vi "Bundle AOL parameters at start.vi"(6 "Case name string":string, 8 "error in (no error)":errorcluster) -> (0 "error out":errorcluster, 2 "cancelled":bool)   [LabVIEW 2013]
uses:
  Typedefs/Imaging Protocols enum.ctl
  Typedefs/AOL modes.ctl
  Global Variables/gl_UI Ctrl Refs.vi
  Global Variables/General Globals.vi
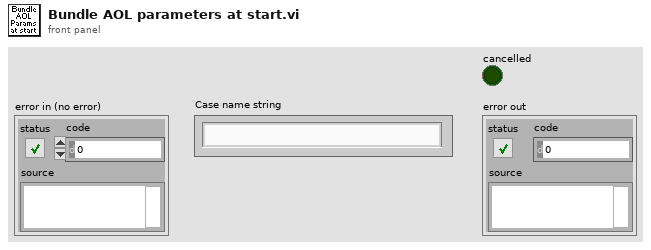
[diagram p1: front panel]
types:
  T1 = typedef "Imaging Protocols enum.ctl" = enum16{"AOL Z-Stack", "Motor Z Stack", "Functional Acquisition", "Single Plane Acquisition", "Volume Acquisition", "Live Imaging", "Live Plane Imaging", "Live Volume Imaging"}
  T2 = typedef "UI ctrl refs cluster.ctl" = cluster{"Top level VI path":path, "Top level VI ref":refnum<vi>, "User menu ref":refnum<k9>, "Sub Panel control":refnum<vi>, "Imaging Param Tab":refnum<vi>, "Occurrence-Start drivers":refnum<k4>, "Occurrence-Speed logging initialised":refnum<k4>, "Occurrence-XYZ stage initialised":refnum<k4>, "Exit button":refnum<vi>, "Status ind":refnum<vi>, "Return to Origin":refnum<vi>, "Speed Logging":refnum<vi>, "Time Lapse":refnum<vi>, "Live Imaging":refnum<vi>, "AOL Z Stack":refnum<vi>, "Motor Z Stack":refnum<vi>, "Funct Acq button":refnum<vi>, "Hard Shutter":refnum<vi>, "Virtual Shutter":refnum<vi>, "Laser Power":refnum<vi>, "AOL Mode":refnum<vi>, "Frame Size":refnum<vi>, "Field of View":refnum<vi>, "Dwell Time":refnum<vi>, "Zoom":refnum<vi>, "AOL Z":refnum<vi>, "Objective":refnum<vi>, "Axis":refnum<vi>, "Paths & Names":refnum<vi>, "Experiment folder path (ind.)":refnum<vi>, "Last State (Ind.)":refnum<vi>, "Laser wavelength ind (nm)":refnum<vi>, "Averages":refnum<vi>, "Angle (degrees)":refnum<vi>, "X centre":refnum<vi>, "Y centre":refnum<vi>, "Plane Mode":refnum<vi>, "# Planes":refnum<vi>, "Z Start":refnum<vi>, "Z Stop":refnum<vi>, "Z Step":refnum<vi>, "PMT 1":refnum<vi>, "PMT 2":refnum<vi>, "Stage XYZ Position":refnum<vi>, "Pockels@Z Start":refnum<vi>, "Pockels@Z Stop":refnum<vi>, "Obtain Z Start":refnum<vi>, "Obtain Z Stop":refnum<vi>, "Live stim.trig.period":refnum<vi>, "Live stim.trig.enable":refnum<vi>, "Funct. Acq. Pockels Modulation":refnum<vi>, "Enable Video Recording":refnum<vi>, "Video Record-Live Imaging":refnum<vi>, "Video Record-Funct acq":refnum<vi>, "AOL Z-stack Chirps Ready (ind)":refnum<vi>, "Center freq ind (nm)":refnum<vi>, "Logging queue (ind)":refnum<vi>, "Back aperture power (ind.)":refnum<vi>, "Power after objective (ind.)":refnum<vi>, "Switch user":refnum<vi>}
  T3 = typedef "AOL_Globals.ctl" = cluster{"Imaging Protocol":T1, "Number of POI":u16, "Number of Miniscans":u16, "Number of Trials":u16, "Number of Cycles ":u64, "# Averaged Frames":u16, "Laser power (%)":u8, "Pockels":dbl, "Acquisition Length (sec)":dbl, "Fill time (us)":dbl, "POI Dwell time (us)":dbl, "Miniscan Dwell time per pixel (us)":dbl, "PMT 1":dbl, "PMT 2":dbl, "Back Apperture":dbl, "Frame Size":T4, "Center Frequency":dbl, "Field of View":dbl, "DwellTime (us)":dbl, "Wavelength (nm)":dbl, "Zoom":dbl, "AOL Z":dbl, "AOL Mode":T5, "GridXY":dbl, "GridZ":dbl, "TriggerPeriod (sec)":dbl, "Number of Pixels in Miniscan":u16, "Experiment folder path":path, "X centre":dbl, "Y centre":dbl, "Angle (degrees)":dbl, "Plane Mode":T6, "Threshold":u16[], "Regenerate Chirps":bool, "Rectangle ROI length (pixels)":u16, "Rectangle ROI height (pixels)":u16, "AOD fill":u16, "Samples Wait after Trigger":u16, "StartUp Delay":i32, "Slip Cycle":u32, "Add Cycle":bool}
  T4 = typedef "Frame Size.ctl" = u16
  T5 = typedef "AOL modes.ctl" = enum16{"Raster", "Structural", "Pointing", "Mini Scan", "Alignment"}
  T6 = typedef "Plane Mode.ctl" = u16
  T7 = typedef "Laser control knob.ctl" = u16
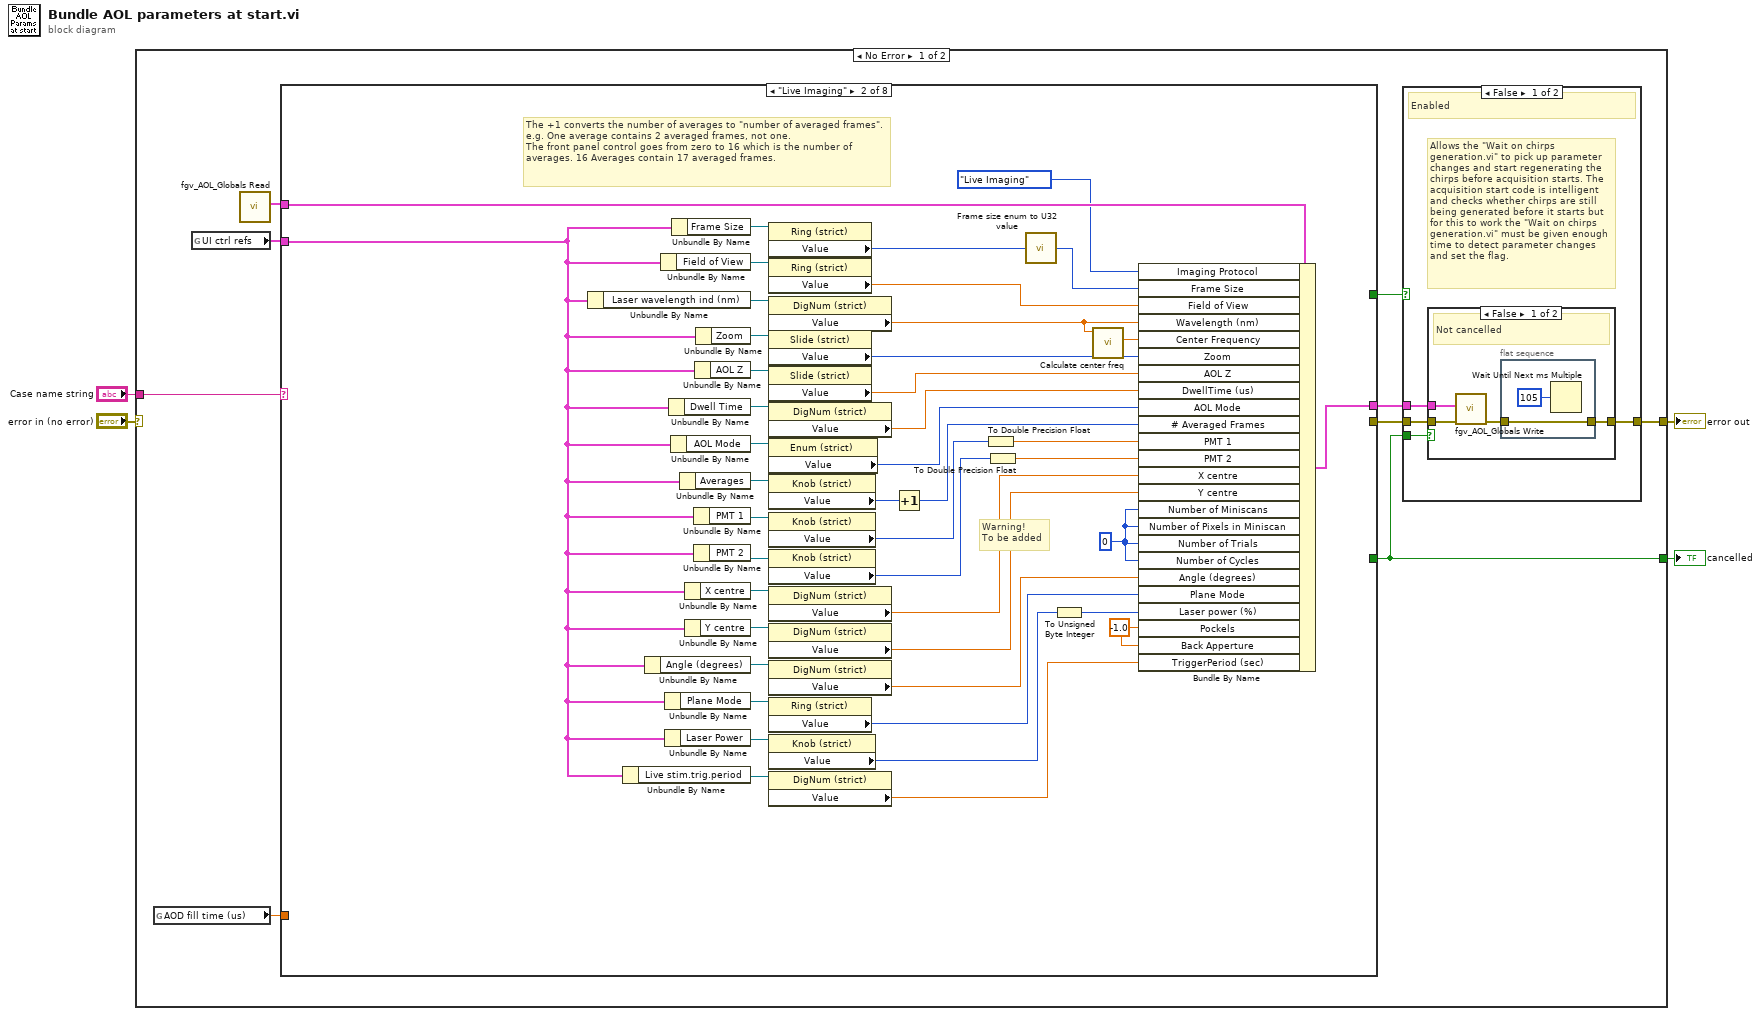
[diagram p0: block diagram]
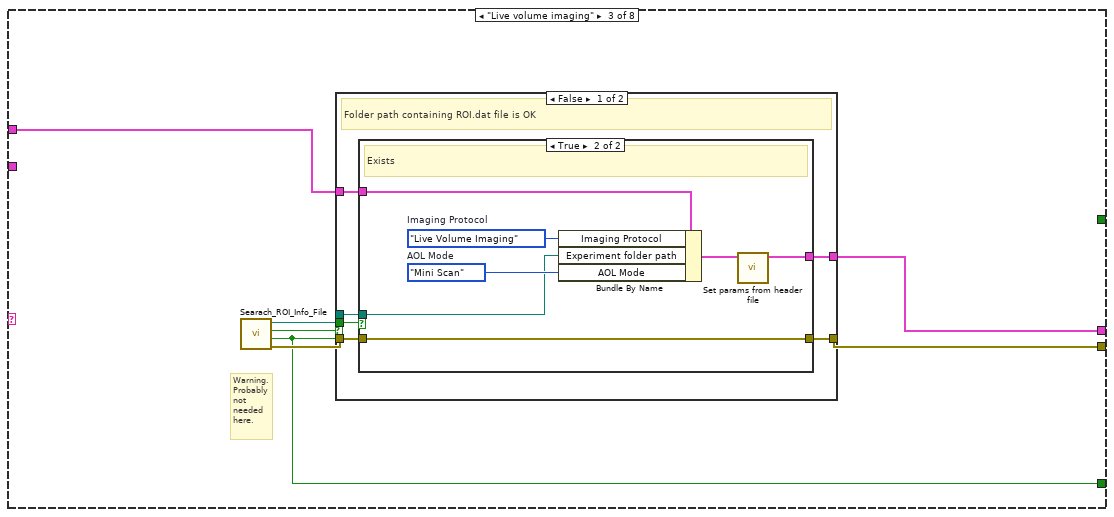
[diagram p5: hidden frame]
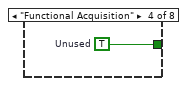
[diagram p8: hidden frame]
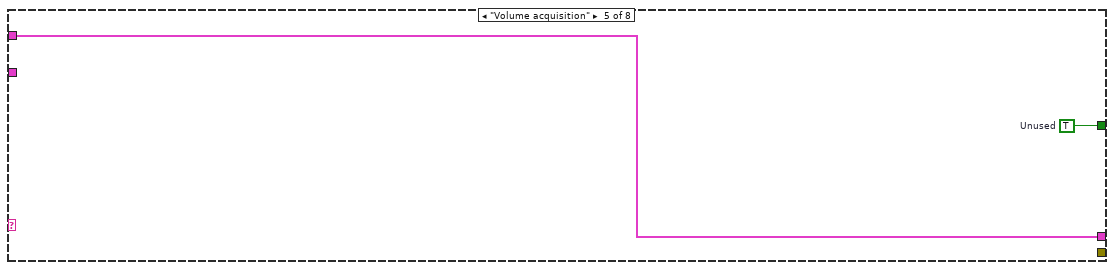
[diagram p9: hidden frame]
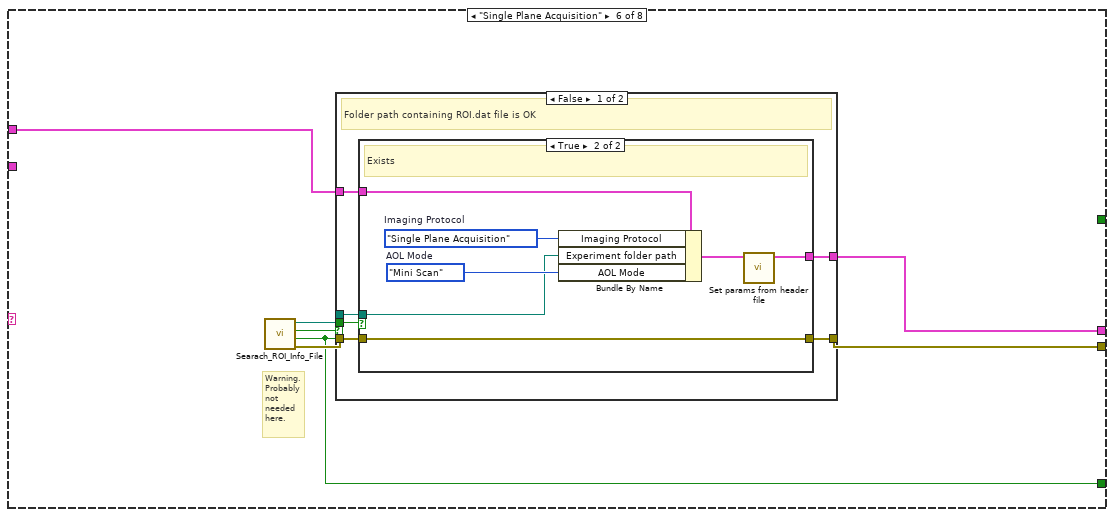
[diagram p10: hidden frame]
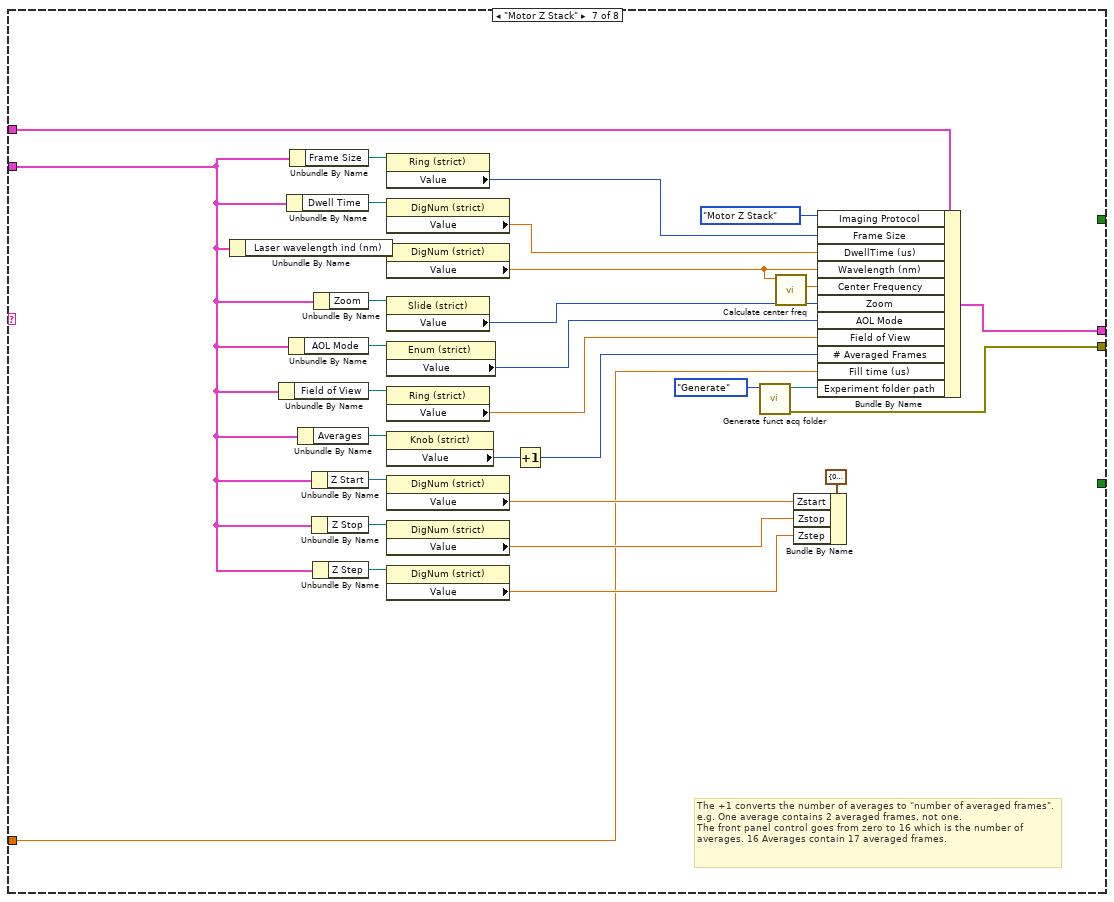
[diagram p13: hidden frame]
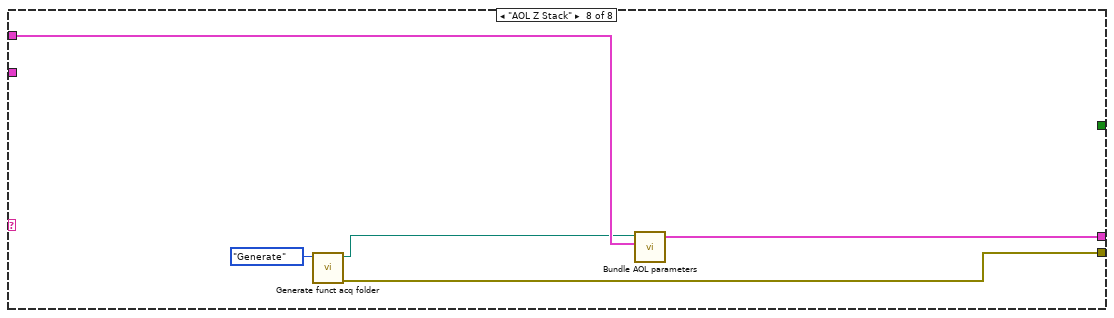
[diagram p14: hidden frame]
diagram:
  n1 = case shown="No Error" "error in (no error)" {
    selector: "error in (no error)" -> [_ w157]
    tunnel: [w13 w157] -> w1
    tunnel: "Case name string" -> [w10 _]
    tunnel: [w6 _] -> w2
    frame No Error {
      n2 = global read "General Globals.vi" "AOD fill time (us)"() -> (w8:dbl)
      n3 = global read "gl_UI Ctrl Refs.vi" "UI ctrl refs"() -> (w9:T2)
      n4 = call "fgv_AOL_Globals Read.vi"() -> ("AOL_Globals"=w11:T3)  [unwired: 9 in, 2 out]
      n5 = case shown="\"Live Imaging\"" w10 {
        tunnel: [w25 w68 w72 _ w96 w99 w126 w154] -> w12
        tunnel: w11 -> [w25 w69 w73 _ w96 w100 w127 w155]
        tunnel: w9 -> [_ w67 _ _ _ _ w128 _]
        tunnel: w8 -> [_ _ _ _ _ _ w123 _]
        tunnel: [_ _ w71 _ _ w98 w125 w153] -> w7
        tunnel: [_ _ w70 _ _ w97 _ _] -> w6
        tunnel: [_ _ _ w94 w95 _ _ _] -> w5
        frame Default {
        }
        frame "Live Imaging" {
          w31 = -1.0 ("Pockels")
          w66 = u16 0 ("Number of Miniscans")
          # "Warning!\nTo be added"
          # "The +1 converts the number of averages to \"number of averaged frames\". e.g. One average contains 2 averaged frames, not one.\nThe front panel control goes from zero to 16 which is the number of averages. 16 Averages contain 17 averaged frames."
          n6 = Unbundle By Name(w67) -> ("Laser wavelength ind (nm)"=w53:refnum<vi>)
          n7 = Unbundle By Name(w67) -> ("Live stim.trig.period"=w30:refnum<vi>)
          n8 = Unbundle By Name(w67) -> ("Angle (degrees)"=w47:refnum<vi>)
          n9 = Unbundle By Name(w67) -> ("Field of View"=w54:refnum<vi>)
          n10 = Unbundle By Name(w67) -> ("Plane Mode"=w44:refnum<vi>)
          n11 = Unbundle By Name(w67) -> ("Laser Power"=w40:refnum<vi>)
          n12 = Unbundle By Name(w67) -> ("Dwell Time"=w50:refnum<vi>)
          n13 = Unbundle By Name(w67) -> ("AOL Mode"=w49:refnum<vi>)
          n14 = Unbundle By Name(w67) -> ("Frame Size"=w55:refnum<vi>)
          n15 = Unbundle By Name(w67) -> ("Averages"=w48:refnum<vi>)
          n16 = Unbundle By Name(w67) -> ("X centre"=w46:refnum<vi>)
          n17 = Unbundle By Name(w67) -> ("Y centre"=w45:refnum<vi>)
          n18 = Unbundle By Name(w67) -> ("PMT 1"=w37:refnum<vi>)
          n19 = Unbundle By Name(w67) -> ("PMT 2"=w36:refnum<vi>)
          n20 = Unbundle By Name(w67) -> ("AOL Z"=w51:refnum<vi>)
          n21 = Unbundle By Name(w67) -> ("Zoom"=w52:refnum<vi>)
          n22 = property on="Property Node" class="Ring (strict)"(reference=w55) -> ("Value"=w42:T4)  [unwired: 1 in, 2 out]
          n23 = property on="Property Node" class="Ring (strict)"(reference=w54) -> ("Value"=w57:sgl)  [unwired: 1 in, 2 out]
          n24 = property on="Property Node" class="DigNum (strict)"(reference=w53) -> ("Value"=w26:dbl)  [unwired: 1 in, 2 out]
          n25 = property on="Property Node" class="Slide (strict)"(reference=w52) -> ("Value"=w61:i8)  [unwired: 1 in, 2 out]
          n26 = property on="Property Node" class="Slide (strict)"(reference=w51) -> ("Value"=w58:sgl)  [unwired: 1 in, 2 out]
          n27 = property on="Property Node" class="DigNum (strict)"(reference=w50) -> ("Value"=w59:dbl)  [unwired: 1 in, 2 out]
          n28 = property on="Property Node" class="Enum (strict)"(reference=w49) -> ("Value"=w65:T5)  [unwired: 1 in, 2 out]
          n29 = property on="Property Node" class="Knob (strict)"(reference=w48) -> ("Value"=w60:u16)  [unwired: 1 in, 2 out]
          n30 = property on="Property Node" class="Knob (strict)"(reference=w37) -> ("Value"=w35:T7)  [unwired: 1 in, 2 out]
          n31 = property on="Property Node" class="Knob (strict)"(reference=w36) -> ("Value"=w34:T7)  [unwired: 1 in, 2 out]
          n32 = property on="Property Node" class="DigNum (strict)"(reference=w46) -> ("Value"=w62:dbl)  [unwired: 1 in, 2 out]
          n33 = property on="Property Node" class="DigNum (strict)"(reference=w45) -> ("Value"=w63:dbl)  [unwired: 1 in, 2 out]
          n34 = property on="Property Node" class="DigNum (strict)"(reference=w47) -> ("Value"=w56:dbl)  [unwired: 1 in, 2 out]
          n35 = property on="Property Node" class="Ring (strict)"(reference=w44) -> ("Value"=w28:T6)  [unwired: 1 in, 2 out]
          n36 = property on="Property Node" class="Knob (strict)"(reference=w40) -> ("Value"=w39:T7)  [unwired: 1 in, 2 out]
          n37 = property on="Property Node" class="DigNum (strict)"(reference=w30) -> ("Value"=w29:dbl)  [unwired: 1 in, 2 out]
          n38 = Increment(x=w60) -> (x+1=w43:u16)
          n39 = To Double Precision Float(number=w35) -> (double precision float=w33:dbl)
          n40 = To Double Precision Float(number=w34) -> (double precision float=w32:dbl)
          n41 = call "Frame size enum to U32 value.vi"("Value"=w42) -> ("Frame Size U32"=w41:u32)
          n42 = To Unsigned Byte Integer(number=w39) -> (unsigned 8bit integer=w38:u8)
          n43 = call "Calculate center freq.vi"("UI Wavelength"=w26) -> ("Centre frequency (MHz)"=w27:dbl)  [unwired: 9 in, 1 out]
          n44 = Bundle By Name(cluster=w69, "Imaging Protocol"=Imaging_Protocols_enum."Live Imaging" ("Imaging Mode"), "Frame Size"=w41, "Field of View"=w57, "Wavelength (nm)"=w26, "Center Frequency"=w27, "Zoom"=w61, "AOL Z"=w58, "DwellTime (us)"=w59, "AOL Mode"=w65, "# Averaged Frames"=w43, "PMT 1"=w33, "PMT 2"=w32, "X centre"=w62, "Y centre"=w63, "Number of Miniscans"=w66, "Number of Pixels in Miniscan"=w66, "Number of Trials"=w66, "Number of Cycles"=w66, "Angle (degrees)"=w56, "Plane Mode"=w28, "Laser power (%)"=w38, "Pockels"=w31, "Back Apperture"=w31, "TriggerPeriod (sec)"=w29) -> (w68:T3)
        }
        frame "Live volume imaging" {
          # "Warning.\nProbably not needed here."
          n45 = call "Searach_ROI_Info_File.vi"() -> ("error out"=w75:errorcluster, "cancelled"=w70:bool, "exists"=w74:bool, "Experiment folder"=w76:path)  [unwired: 8 in]
          n46 = case shown="False" w70 {
            tunnel: w76 -> [w82 _]
            tunnel: w75 -> [w81 w92]
            tunnel: w74 -> [w80 _]
            tunnel: w73 -> [w79 w93]
            tunnel: [w78 w93] -> w72
            tunnel: [w77 w92] -> w71
            frame False {
              # "Folder path containing ROI.dat file is OK"
              n47 = case shown="True" w80 {
                tunnel: w82 -> [_ w89]
                tunnel: w81 -> [w84 w86]
                tunnel: w79 -> [w83 w88]
                tunnel: [w83 w85] -> w78
                tunnel: [w84 w86] -> w77
                frame False {
                  # "Deos not exist"
                }
                frame True {
                  w90 = AOL_modes."Mini Scan"  # AOL Mode
                  w91 = Imaging_Protocols_enum."Live Volume Imaging"  # Imaging Protocol
                  # "Exists"
                  n48 = Bundle By Name(cluster=w88, "Imaging Protocol"=w91, "Experiment folder path"=w89, "AOL Mode"=w90) -> (w87:T3)
                  n49 = call "Set params from header file.vi"("AOL_Globals in"=w87) -> ("AOL_Globals out"=w85:T3)  [unwired: 10 in]
                }
              }
            }
            frame True {
              # "Cancelled"
            }
          }
        }
        frame "Functional Acquisition" {
          w94 = TRUE  # Unused
        }
        frame "Volume acquisition" {
          w95 = TRUE  # Unused
        }
        frame "Single Plane Acquisition" {
          # "Warning.\nProbably not needed here."
          n50 = call "Searach_ROI_Info_File.vi"() -> ("error out"=w102:errorcluster, "cancelled"=w97:bool, "exists"=w101:bool, "Experiment folder"=w103:path)  [unwired: 8 in]
          n51 = case shown="False" w97 {
            tunnel: w103 -> [w109 _]
            tunnel: w102 -> [w108 w119]
            tunnel: w101 -> [w107 _]
            tunnel: w100 -> [w106 w120]
            tunnel: [w105 w120] -> w99
            tunnel: [w104 w119] -> w98
            frame False {
              # "Folder path containing ROI.dat file is OK"
              n52 = case shown="True" w107 {
                tunnel: w109 -> [_ w116]
                tunnel: w108 -> [w111 w114]
                tunnel: w106 -> [w110 w115]
                tunnel: [w110 w112] -> w105
                tunnel: [w111 w114] -> w104
                frame False {
                  # "Deos not exist"
                }
                frame True {
                  w117 = AOL_modes."Mini Scan"  # AOL Mode
                  w118 = Imaging_Protocols_enum."Single Plane Acquisition"  # Imaging Protocol
                  # "Exists"
                  n53 = Bundle By Name(cluster=w115, "Imaging Protocol"=w118, "Experiment folder path"=w116, "AOL Mode"=w117) -> (w113:T3)
                  n54 = call "Set params from header file.vi"("AOL_Globals in"=w113) -> ("AOL_Globals out"=w112:T3)  [unwired: 10 in]
                }
              }
            }
            frame True {
              # "Cancelled"
            }
          }
        }
        frame "Motor Z Stack" {
          # "The +1 converts the number of averages to \"number of averaged frames\". e.g. One average contains 2 averaged frames, not one.\nThe front panel control goes from zero to 16 which is the number of averages. 16 Averages contain 17 averaged frames."
          n55 = Unbundle By Name(w128) -> ("Laser wavelength ind (nm)"=w143:refnum<vi>)
          n56 = Unbundle By Name(w128) -> ("Field of View"=w141:refnum<vi>)
          n57 = Unbundle By Name(w128) -> ("Dwell Time"=w145:refnum<vi>)
          n58 = Unbundle By Name(w128) -> ("AOL Mode"=w142:refnum<vi>)
          n59 = Unbundle By Name(w128) -> ("Frame Size"=w147:refnum<vi>)
          n60 = Unbundle By Name(w128) -> ("Averages"=w140:refnum<vi>)
          n61 = Unbundle By Name(w128) -> ("Z Start"=w133:refnum<vi>)
          n62 = Unbundle By Name(w128) -> ("Z Stop"=w134:refnum<vi>)
          n63 = Unbundle By Name(w128) -> ("Z Step"=w135:refnum<vi>)
          n64 = Unbundle By Name(w128) -> ("Zoom"=w144:refnum<vi>)
          n65 = property class="Ring (strict)"(reference=w147) -> ("Value"=w146:u16)  [unwired: 1 in, 2 out]
          n66 = property class="DigNum (strict)"(reference=w145) -> ("Value"=w139:dbl)  [unwired: 1 in, 2 out]
          n67 = property class="DigNum (strict)"(reference=w143) -> ("Value"=w122:dbl)  [unwired: 1 in, 2 out]
          n68 = property class="Slide (strict)"(reference=w144) -> ("Value"=w132:i8)  [unwired: 1 in, 2 out]
          n69 = property class="Enum (strict)"(reference=w142) -> ("Value"=w138:T5)  [unwired: 1 in, 2 out]
          n70 = property class="Ring (strict)"(reference=w141) -> ("Value"=w137:sgl)  [unwired: 1 in, 2 out]
          n71 = property class="Knob (strict)"(reference=w140) -> ("Value"=w136:u16)  [unwired: 1 in, 2 out]
          n72 = property class="DigNum (strict)"(reference=w133) -> ("Value"=w131:dbl)  [unwired: 1 in, 2 out]
          n73 = property class="DigNum (strict)"(reference=w134) -> ("Value"=w130:dbl)  [unwired: 1 in, 2 out]
          n74 = property class="DigNum (strict)"(reference=w135) -> ("Value"=w129:dbl)  [unwired: 1 in, 2 out]
          n75 = Increment(x=w136) -> (x+1=w124:u16)
          n76 = call "Generate funct acq folder.vi"("Function"=enum16{"Generate", "Obtain"}."Generate") -> ("error out"=w125:errorcluster, "Funct acq experiment folder path"=w148:path)  [unwired: 9 in]
          n77 = call "Calculate center freq.vi"("UI Wavelength"=w122) -> ("Centre frequency (MHz)"=w121:dbl)  [unwired: 9 in, 1 out]
          n78 = Bundle By Name(cluster=cluster{"Zstart":dbl, "Zstop":dbl, "Zstep":dbl} {"Zstart"=0.0, "Zstop"=0.0, "Zstep"=0.0} ("ZStack"), "Zstart"=w131, "Zstop"=w130, "Zstep"=w129) -> ()  [unwired: 1 out]
          n79 = Bundle By Name(cluster=w127, "Imaging Protocol"=Imaging_Protocols_enum."Motor Z Stack" ("Imaging Mode"), "Frame Size"=w146, "DwellTime (us)"=w139, "Wavelength (nm)"=w122, "Center Frequency"=w121, "Zoom"=w132, "AOL Mode"=w138, "Field of View"=w137, "# Averaged Frames"=w124, "Fill time (us)"=w123, "Experiment folder path"=w148) -> (w126:T3)
        }
        frame "AOL Z Stack" {
          n80 = call "Generate funct acq folder.vi"("Function"=enum16{"Generate", "Obtain"}."Generate") -> ("error out"=w153:errorcluster, "Funct acq experiment folder path"=w152:path)  [unwired: 9 in]
          n81 = call "Bundle AOL parameters.vi"("AOL_Globals in"=w155, "Experiment folder path"=w152) -> ("AOL_Globals out"=w154:T3)  [unwired: 9 in]
        }
      }
      n82 = case shown="False" w5 {
        tunnel: [w17 _] -> w13
        tunnel: w12 -> [w16 _]
        tunnel: w7 -> [w15 _]
        tunnel: w6 -> [w14 _]
        frame False {
          # "Allows the\t\"Wait on chirps generation.vi\" to pick up parameter changes and start regenerating the chirps before acquisition starts. The acquisition start code is intelligent and checks whether chirps are still being generated before it starts but for this to work the \"Wait on chirps generation.vi\" must be given enough time to detect parameter changes and set the flag."
          # "Enabled"
          n83 = case shown="False" w14 {
            tunnel: [w18 w24] -> w17
            tunnel: w16 -> [w21 _]
            tunnel: w15 -> [w20 w24]
            frame False {
              # "Not cancelled"
              n84 = call "fgv_AOL_Globals Write.vi"("error in (no error)"=w20, "AOL_Globals"=w21) -> ("error out"=w19:errorcluster)  [unwired: 9 in]
              n85 = flat-sequence {
                tunnel: w19 -> [w23]
                tunnel: [w23] -> w18
                frame #0 {
                  n86 = Wait Until Next ms Multiple(millisecond multiple=u32 105) -> ()  [unwired: 1 out]
                }
              }
            }
            frame True {
              # "Cancelled"
            }
          }
        }
        frame True {
          # "Unused"
        }
      }
    }
    frame Error {
    }
  }
  "error out" <- w1
  "cancelled" <- w2
